vi "Read Analogue.vi"(8 "error in (no error)":errorcluster, 11 "PS in":refnum<class "Keysight 6700C.lvclass">) -> (0 "error out":errorcluster, 2 "Measurements":dbl, 3 "PS out":refnum<class "Keysight 6700C.lvclass">)   [LabVIEW 2021, in "Concrete.lvlib" / "Keysight 6700C.lvclass"]
uses:
  Keysight 6700C.lvclass
  Keysight 6700C.lvclass/Keysight 6700C.ctl
  Harware Abstraction/AnalogIO/Power Supply.lvclass
  <instrlib>/Agilent N6700 Series/Agilent N6700 Series.lvlib
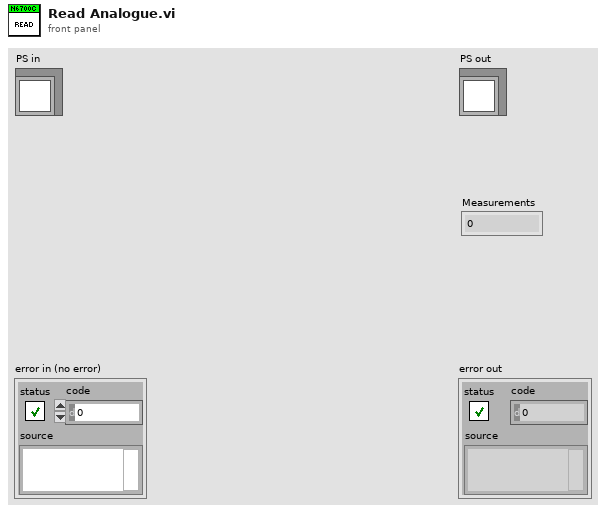
[diagram p1: front panel]
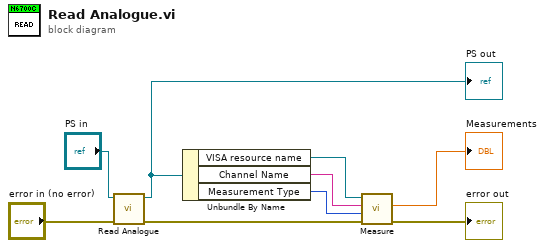
[diagram p0: block diagram]
diagram:
  n1 = call-parent "Read Analogue.vi"("error in (no error)"="error in (no error)", "PS in"="PS in") -> ("error out"=w7:errorcluster, "PS out"=w5:refnum<class "Keysight 6700C.lvclass">)  [unwired: 7 in, 1 out]
  "PS out" <- w5
  n2 = Unbundle By Name(w5) -> ("VISA resource name"=w4:refnum<visa-resource-name>, "Channel Name"=w2:string, "Measurement Type"=w1:i32)
  n3 = call <instrlib>:"Measure.vi"("error in (no error)"=w7, "Measurement Type (1: Voltage)"=w1, "Channel Name (1)"=w2, "VISA resource name"=w4) -> ("error out"=→"error out":errorcluster, "Measurement"=→"Measurements":dbl)  [unwired: 5 in, 1 out]
